vi "rvc 3D Axis Quaternion.vi"(10 "translation vector":dbl[](array[numeric])=[0.0, 0.0, 0.0], 11 "quaternion":T1) -> (3 "SceneNode out":refnum<vi>(3d-picture))   [LabVIEW 2017]
uses:
  <vilib>/robotics/Kinematics/Quaternion.ctl
  <vilib>/Analysis/baseanly.llb/Outer Product.vi
  <vilib>/Analysis/baseanly.llb/Real Outer Product.vi
  <vilib>/robotics/Kinematics/Create Lie Group Matrix.vi
  <vilib>/Analysis/Matrix/Numeric/Multiply/Multiply.vi
  <vilib>/Analysis/Matrix/Numeric/Multiply/Multiply - RM,R.vi
  <vilib>/Analysis/Matrix/Numeric/Multiply/Multiply - R,RM.vi
  <vilib>/Analysis/Matrix/Numeric/Add/Add.vi
  <vilib>/Analysis/Matrix/Numeric/Add/Add - RM,RM.vi
  <vilib>/robotics/Kinematics/NI_Kinematics.lvlib
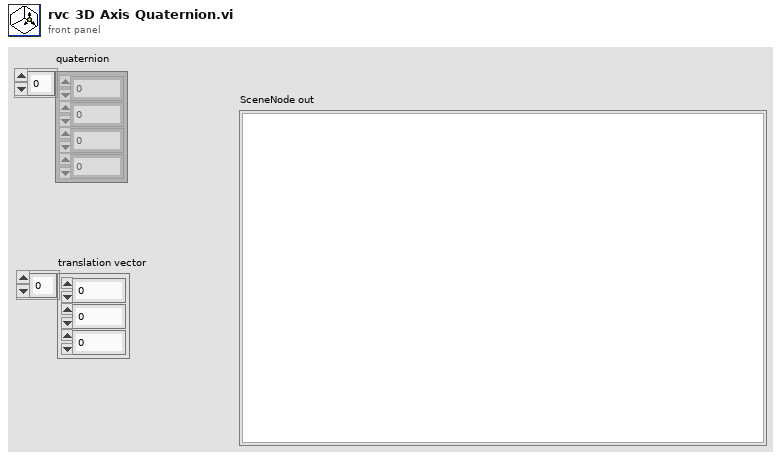
[diagram p1: front panel]
types:
  T1 = typedef "NI_Kinematics.lvlib/Quaternion.ctl" = dbl[]
  T2 = typedef "NI_Matrix.lvlib/RealMatrix.ctl" = dbl[][]
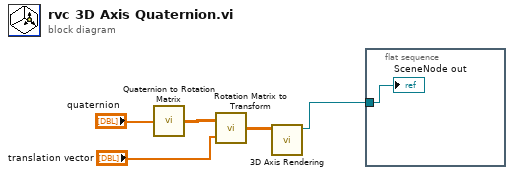
[diagram p0: block diagram]
diagram:
  n1 = call <vilib>:"Quaternion to Rotation Matrix.vi"("quaternion"="quaternion") -> ("rotation matrix"=w3:T2)
  n2 = call <vilib>:"Rotation Matrix to Transform.vi"("translation vector"="translation vector", "rotation matrix"=w3) -> ("transform"=w2:T2)
  n3 = call "3D Axis Rendering.vi"("rotation matrix"=w2) -> ("SceneNode out"=w5:refnum<vi>)  [unwired: 10 in]
  n4 = flat-sequence {
    tunnel: w5 -> [w6]
    frame #0 {
      "SceneNode out" <- w6
    }
  }
